vi "Read Payload.vi"(8 "error in":errorcluster, 11 "ChanMngOOB_Tx in":refnum<class "ChnMngOOB_Tx.lvclass">) -> (0 "error out":errorcluster, 2 "data":T1, 3 "ChanMngOOB_Tx out":refnum<class "ChnMngOOB_Tx.lvclass">)   [LabVIEW 2021, in "ChnMngOOB_Tx.lvclass"]
uses:
  ChnMngOOB_Tx.lvclass
  C:/Program Files/National Instruments/LabVIEW 2021/vi.lib/CIF Foundation/CIF Out of Band Commands/CIFOutOfBand.lvclass
  Typedef/Template Payload.ctl
  typedef/Channel List for OOB.ctl
  <vilib>/CIF Foundation/CIF Channels Core/CIFChannels/Typedef/Direction.ctl
  Typedef/FIFO Publisher Return.ctl
  <vilib>/CIF Foundation/CIF Out of Band Commands/CIFOutOfBand.lvclass/CIFOutOfBand.ctl
  <vilib>/CIF Foundation/CIF Out of Band Commands/CIFOutOfBand.lvclass
  <vilib>/CIF Foundation/CIF Channels Core/CIFChannels/CIFChannels.lvclass
  CIFChannelMng.lvclass
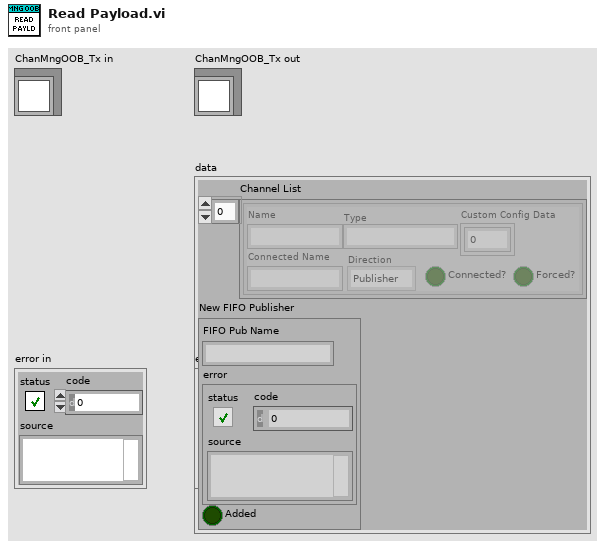
[diagram p1: front panel]
types:
  T1 = typedef "ChnMngOOB_Tx.lvclass/Template Payload.ctl" = cluster{"Channel List":T2[], "New FIFO Publisher":T4}
  T2 = typedef "CIFChannelMng.lvclass/Channel List for OOB.ctl" = cluster{"Name":string, "Direction":T3, "Type":string, "Connected?":bool, "Connected Name":string, "Custom Config Data":u8[], "Forced?":bool}
  T3 = typedef "CIFChannels.lvclass/Direction.ctl" = enum16{"Publisher", "Subscriber"}
  T4 = typedef "ChnMngOOB_Tx.lvclass/FIFO Publisher Return.ctl" = cluster{"FIFO Pub Name":string, "error":errorcluster, "Added":bool}
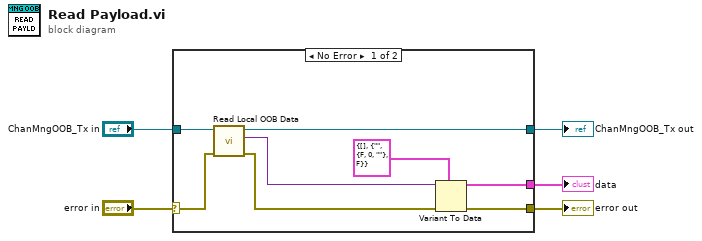
[diagram p0: block diagram]
diagram:
  n1 = case shown="No Error" "error in" {
    selector: "error in" -> [w12 w15]
    tunnel: [w11 w15] -> w5
    tunnel: [w8 w14] -> w4
    tunnel: "ChanMngOOB_Tx in" -> [w13 w14]
    tunnel: [w7 _] -> w1
    frame No Error {
      n2 = call <vilib>:"Read Local OOB Data.vi"("error in"=w12, "OOB in"=w13) -> ("error out"=w10:errorcluster, "Local OOB Data"=w9:variant, "OOB out"=w8:refnum<class "ChnMngOOB_Tx.lvclass">)  [unwired: 7 in]
      n3 = Variant To Data(error in=w10, type=T1 {"Channel List"=[], "New FIFO Publisher"={"FIFO Pub Name"="", "error"={"status"=FALSE, "code"=0, "source"=""}, "Added"=FALSE}} ("Template Payload"), Variant=w9) -> (data=w7:T1, error out=w11:errorcluster)
    }
    frame Error {
    }
  }
  "error out" <- w5
  "ChanMngOOB_Tx out" <- w4
  "data" <- w1
